vi "Simulador RLC - Versão Final - Renan_Nunes-Cardoso_Martins.vi"() -> ()   [LabVIEW 2020]
uses:
  <vilib>/Utility/file.llb/Read Delimited Spreadsheet (DBL).vi
  <vilib>/measure/NI_MABase.lvlib
panel:
  in  "?":bool
  out "?":bool
  in  "?":bool
  in  "?":u16(ring) items=["Onda Quadrada", "Onda Senoidal", "Inserir Onda"]
  in  "Plota Voltagem":bool
  in  "Plota Corrente":bool
  out "Este é um parâmetro \nescondido, serve para \nmostrar o Delta T do \narquivo insderido:":dbl
  in  "Arquivo texto da onda":path
  out "ONDA DE ENTRADA e \nVOLTAGEM NO CAPACITOR":dbl[][](graph)
  out "ONDA DE ENTRADA e CORRENTE":dbl[][](graph)
  in  "?":T1={"Taxa de Amostragem"=1000.0, "Número de amostras"=1000.0} {"Número de amostras" format="%#.6g"; "Taxa de Amostragem" format="%#.6g"}
  in  "C - Capacitância":dbl min=0.0
  in  "L -  Indutância":dbl min=0.0
  in  "R - Resistência":dbl min=0.0
  in  "Amplitude":dbl min=0.0
  in  "Duty Cicle":dbl min=0.0
  in  "Frequência":dbl min=0.0
  # "SIMULADOR RLC"
  # "LIGA/DESLIGA"
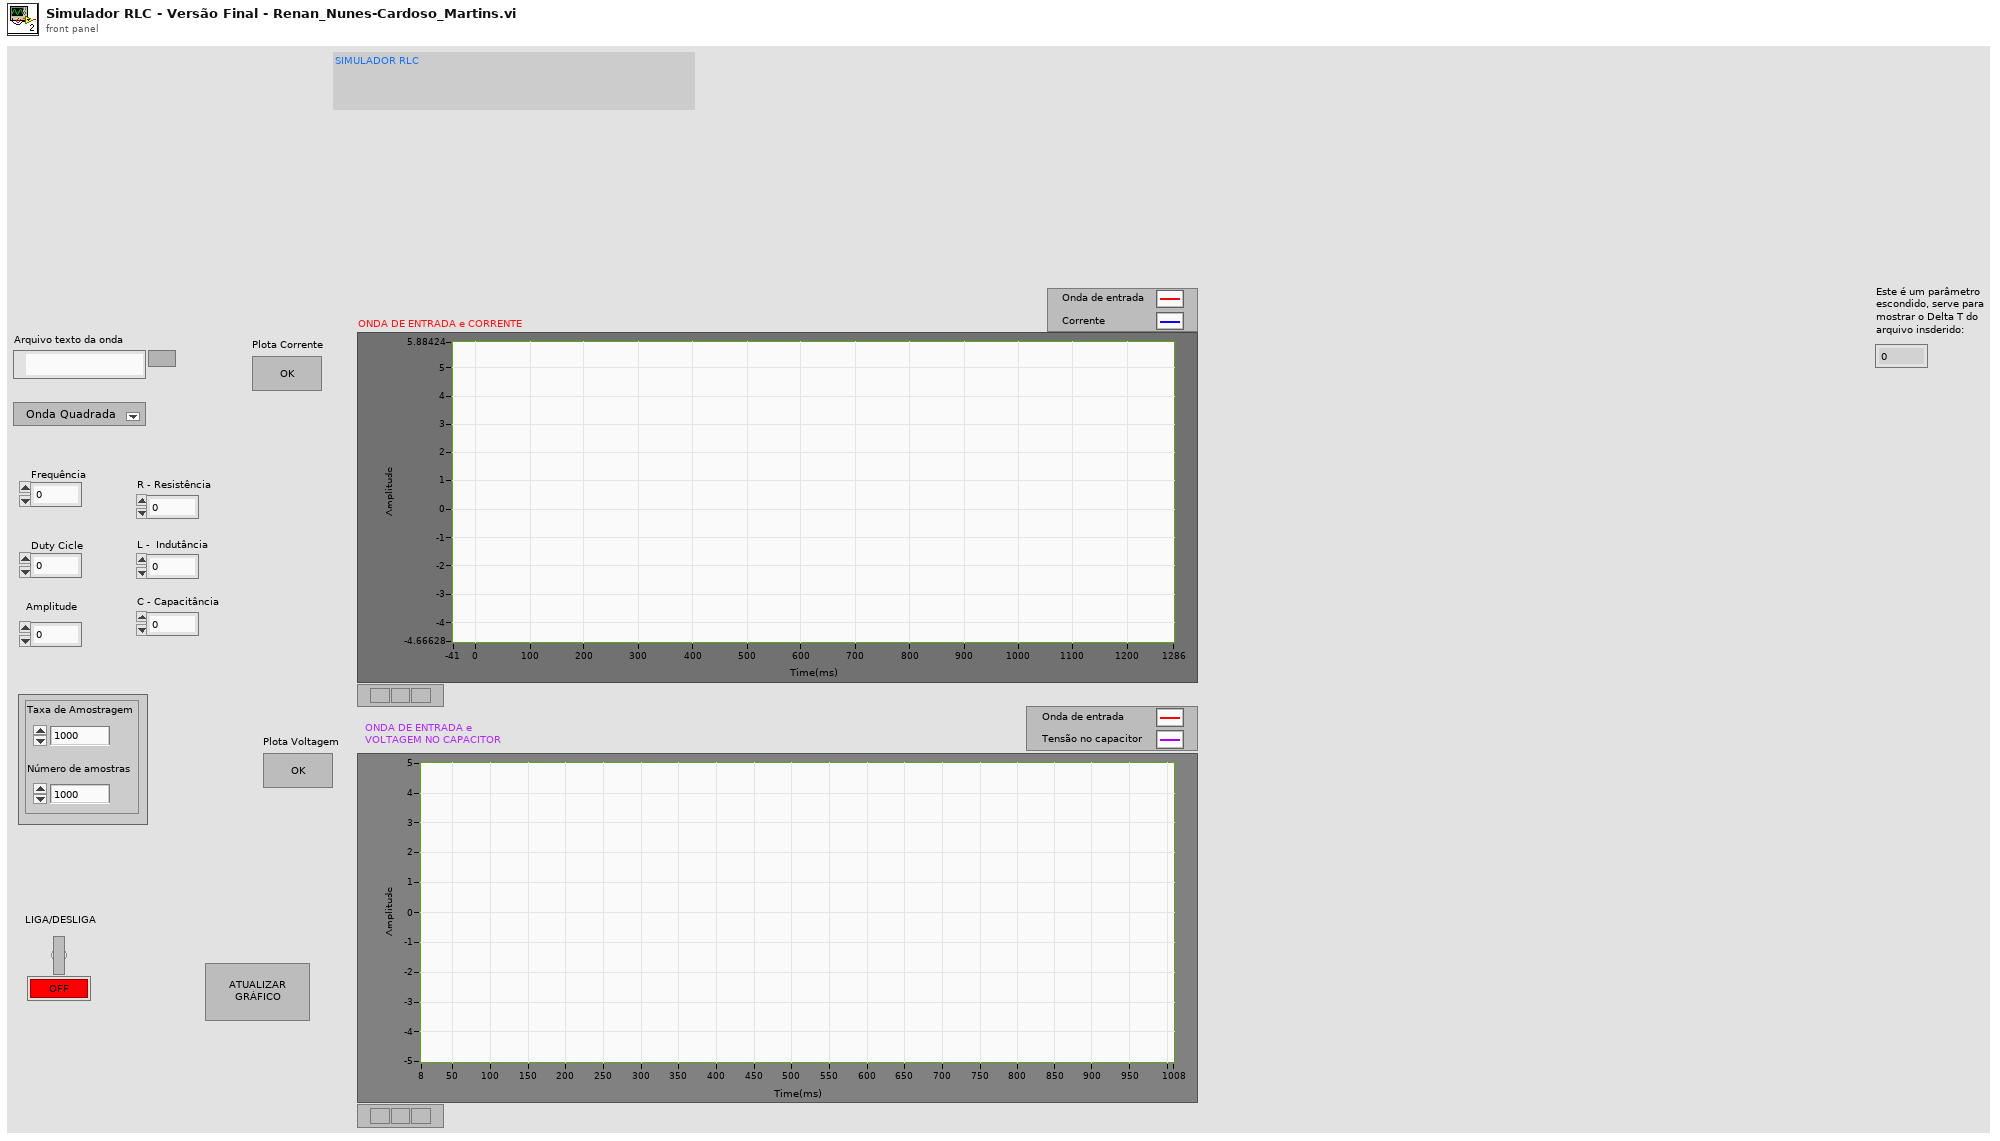
[diagram p1: front panel]
types:
  T1 = cluster{"Taxa de Amostragem":dbl, "Número de amostras":dbl}
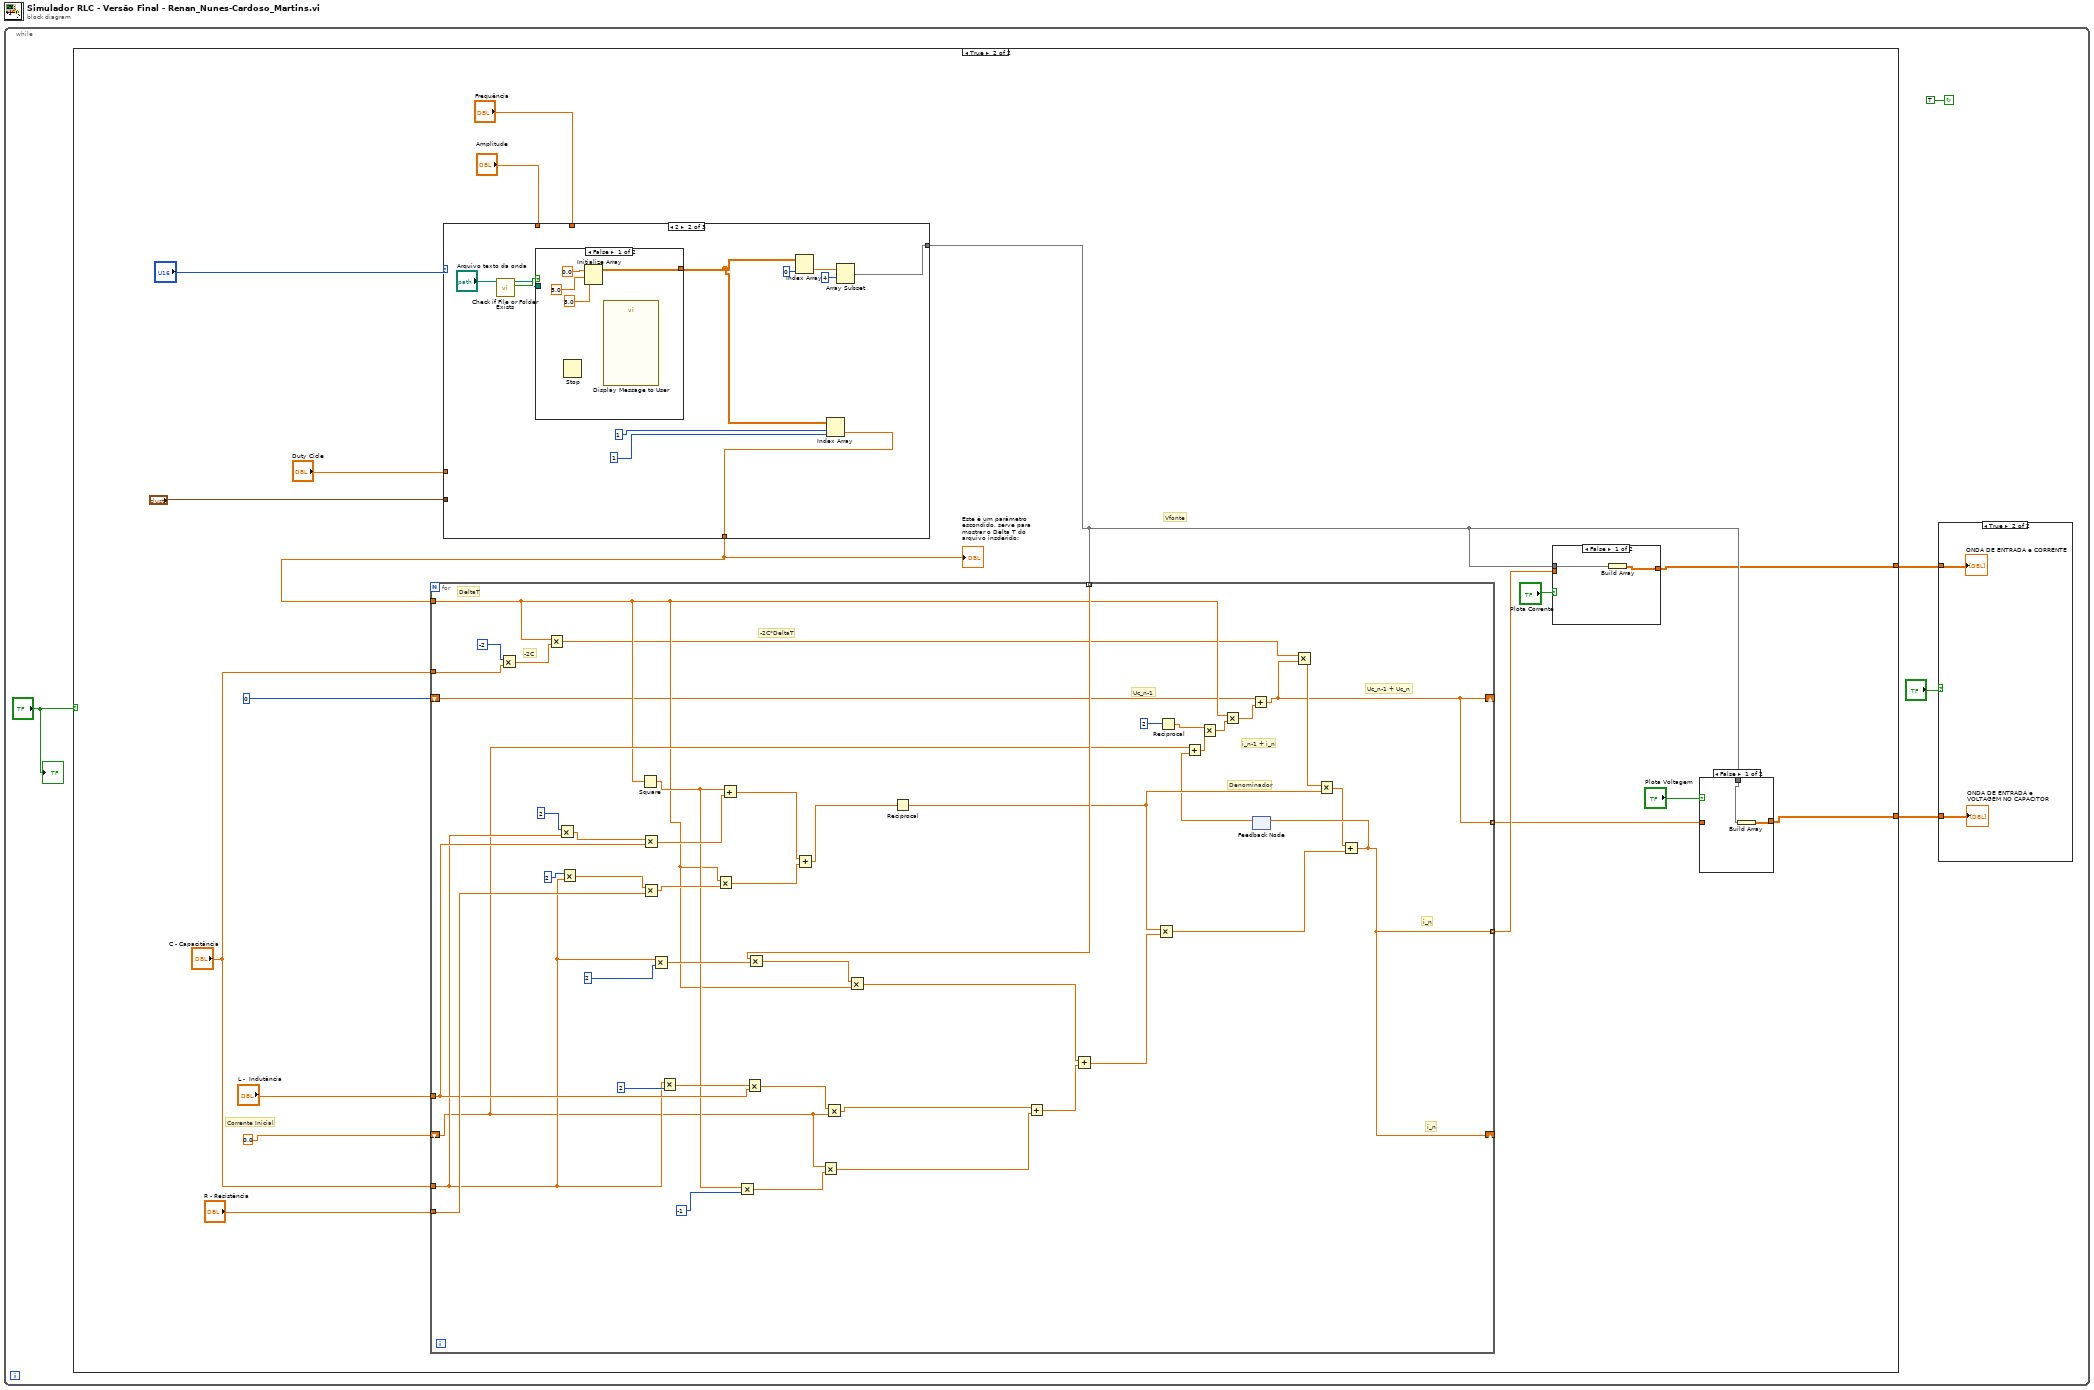
[diagram p0: block diagram]
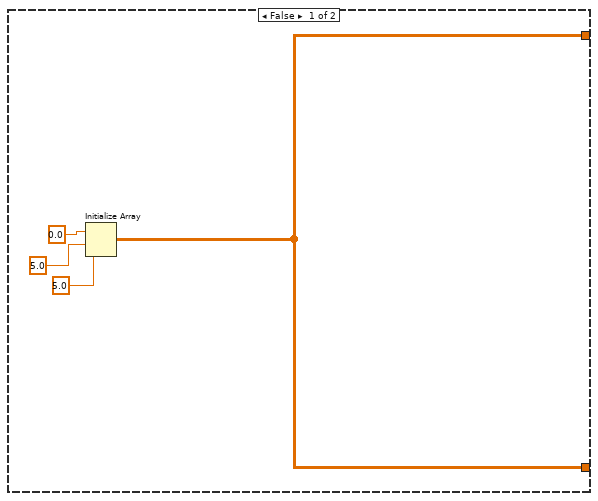
[diagram p3: hidden frame]
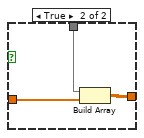
[diagram p4: hidden frame]
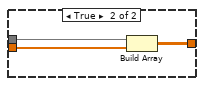
[diagram p5: hidden frame]
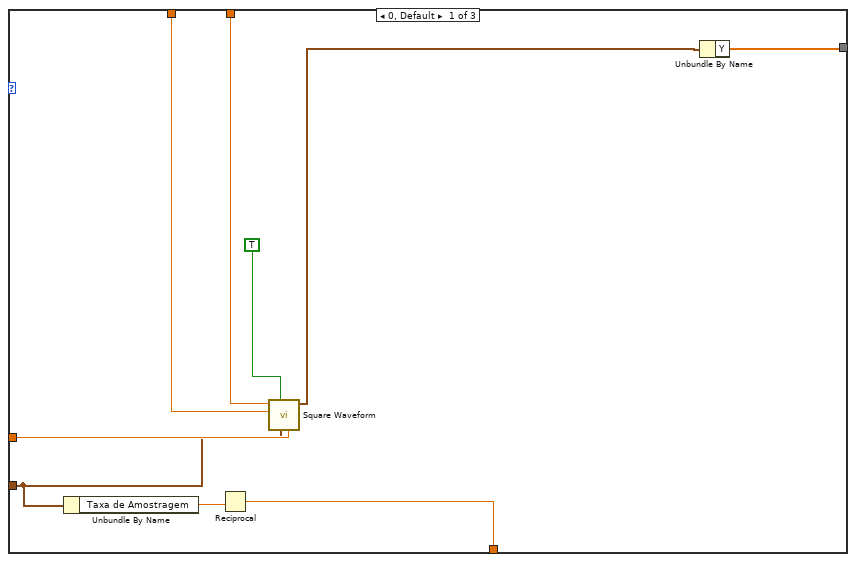
[diagram p6: hidden frame]
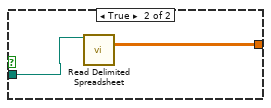
[diagram p7: hidden frame]
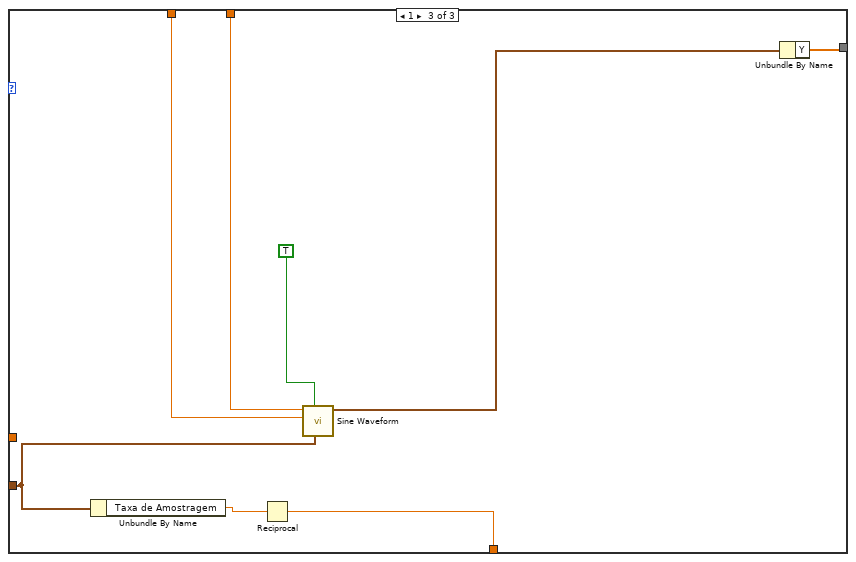
[diagram p8: hidden frame]
diagram:
  n1 = while {
    stop <- TRUE continue-if-true
    n2 = case shown="True" "?" {
      tunnel: [w8 w13] -> w3
      tunnel: [w8 w12] -> w2
      frame False {
        n3 = Initialize Array(0.0 ("element"), 5.0 ("element"), 5.0 ("element")) -> (w8:dbl[][])
      }
      frame True {
        # "Vfonte"
        # "Corrente Inicial"
        n4 = case shown="2" "?" {
          tunnel: "Amplitude" -> [w94 _ w118]
          tunnel: "Frequência" -> [w93 _ w119]
          tunnel: "Duty Cicle" -> [w92 _ _]
          tunnel: [w89 w102 w115] -> w19
          tunnel: "?" -> [w87 _ w114]
          tunnel: [w86 w98 w112] -> w17
          frame 0, Default {
            n5 = Unbundle By Name(w87) -> ("Taxa de Amostragem"=w88:dbl)
            n6 = Reciprocal(x=w88) -> (1/x=w86:dbl)
            n7 = call <vilib>:"Square Waveform.vi"("duty cycle (%)"=w92, "sampling info"=w87, "reset signal"=TRUE, "amplitude"=w94, "frequency"=w93) -> ("signal out"=w90:waveform(dbl))  [unwired: 5 in, 1 out]
            n8 = Unbundle By Name(w90) -> ("Y"=w89:dbl[])
          }
          frame 2 {
            n9 = call <vilib>:"Check if File or Folder Exists.vi"("path"="Arquivo texto da onda") -> ("file or folder exists?"=w96:bool, "dup path"=w95:path)  [unwired: 8 in, 1 out]
            n10 = case shown="False" w96 {
              tunnel: [w109 w111] -> w100
              tunnel: w95 -> [_ w110]
              frame False {
                n11 = Stop() -> ()  [unwired: 1 in]
                n12 = Initialize Array(0.0 ("element"), 5.0 ("element"), 5.0 ("element")) -> (w109:dbl[][])
                n13 = call "Display Message to User"() -> ()  [unwired: 10 in, 2 out]
              }
              frame True {
                n14 = call-poly <vilib>:"Read Delimited Spreadsheet.vi"("file path (dialog if empty)"=w110) -> ("all rows"=w111:dbl[][])  [unwired: 9 in, 5 out]
              }
            }
            n15 = Index Array(array=w100, index (col)=0 ("disabled index (col)")) -> (element=w103:dbl[])  [unwired: 1 in]
            n16 = Index Array(array=w100, index (row)=1 ("disabled index (col)"), index (col)=1 ("disabled index (col)")) -> (element=w98:dbl)
            n17 = Array Subset(array=w103, index=4) -> (w102:dbl[])  [unwired: 1 in]
          }
          frame 1 {
            n18 = Unbundle By Name(w114) -> ("Taxa de Amostragem"=w113:dbl)
            n19 = Reciprocal(x=w113) -> (1/x=w112:dbl)
            n20 = call <vilib>:"Sine Waveform.vi"("sampling info"=w114, "reset signal"=TRUE, "amplitude"=w118, "frequency"=w119) -> ("signal out"=w116:waveform(dbl))  [unwired: 6 in, 1 out]
            n21 = Unbundle By Name(w116) -> ("Y"=w115:dbl[])
          }
        }
        "Este é um parâmetro \nescondido, serve para \nmostrar o Delta T do \narquivo insderido:" <- w17
        n22 = for {
          tunnel: w19 -> [w76] mode=indexing
          tunnel: w17 -> [w50]
          tunnel: [w42] -> w21 mode=indexing
          shift-right: [w42] -> _
          shift-left: 0.0 -> [w55]
          tunnel: "R - Resistência" -> [w63]
          tunnel: "L -  Indutância" -> [w62]
          tunnel: "C - Capacitância" -> [w61]
          tunnel: "C - Capacitância" -> [w58]
          shift-right: [w40] -> _
          shift-left: 0 -> [w48]
          tunnel: [w40] -> w20 mode=indexing
          # "Uc_n-1"
          # "-2C*DeltaT"
          # "-2C"
          # "Denominador"
          # "DeltaT"
          # "i_n"
          # "i_n"
          # "Uc_n-1 + Uc_n"
          # "i_n-1 + i_n"
          n23 = Multiply(x=-2, y=w58) -> (x*y=w56:dbl)
          n24 = Multiply(x=w50, y=w56) -> (x*y=w47:dbl)
          n25 = Multiply(x=2, y=w61) -> (x*y=w84:dbl)
          n26 = Multiply(x=2, y=w61) -> (x*y=w81:dbl)
          n27 = Square(x=w50) -> (x^2=w59:dbl)
          n28 = Multiply(x=w84, y=w62) -> (x*y=w83:dbl)
          n29 = Multiply(x=w81, y=w63) -> (x*y=w80:dbl)
          n30 = Multiply(x=w61, y=2) -> (x*y=w75:dbl)
          n31 = Multiply(x=w61, y=2) -> (x*y=w72:dbl)
          n32 = Multiply(x=w50, y=w80) -> (x*y=w78:dbl)
          n33 = Add(x=w59, y=w83) -> (x+y=w79:dbl)
          n34 = Multiply(x=w59, y=-1) -> (x*y=w67:dbl)
          n35 = Multiply(x=w72, y=w62) -> (x*y=w66:dbl)
          n36 = Multiply(x=w76, y=w75) -> (x*y=w74:dbl)
          n37 = Add(x=w79, y=w78) -> (x+y=w69:dbl)
          n38 = Multiply(x=w55, y=w67) -> (x*y=w64:dbl)
          n39 = Multiply(x=w66, y=w55) -> (x*y=w65:dbl)
          n40 = Multiply(x=w74, y=w50) -> (x*y=w71:dbl)
          n41 = Reciprocal(x=w69) -> (1/x=w46:dbl)
          n42 = Add(x=w65, y=w64) -> (x+y=w70:dbl)
          n43 = Add(x=w71, y=w70) -> (x+y=w68:dbl)
          n44 = Multiply(x=w46, y=w68) -> (x*y=w44:dbl)
          n45 = Reciprocal(x=2) -> (1/x=w53:dbl)
          n46 = feedback #1() -> (w43:dbl)  [unwired: 1 in]
          n47 = Add(x=w55, y=w43) -> (x+y=w52:dbl)
          n48 = Multiply(x=w53, y=w52) -> (x*y=w51:dbl)
          n49 = Multiply(x=w50, y=w51) -> (x*y=w49:dbl)
          n50 = Add(x=w48, y=w49) -> (x+y=w40:dbl)
          n51 = Multiply(x=w47, y=w40) -> (x*y=w45:dbl)
          n52 = Multiply(x=w45, y=w46) -> (x*y=w41:dbl)
          n53 = Add(x=w41, y=w44) -> (x+y=w42:dbl)
          n54 = feedback-in #1(w42) -> ()
        }
        n55 = case shown="False" "Plota Corrente" {
          tunnel: [w35 w39] -> w12
          tunnel: w21 -> [_ w38]
          tunnel: w19 -> [w36 w37]
          frame False {
            n56 = Build Array(w36) -> (w35:dbl[][])
          }
          frame True {
            n57 = Build Array(w37, w38) -> (w39:dbl[][])
          }
        }
        n58 = case shown="False" "Plota Voltagem" {
          tunnel: [w30 w34] -> w13
          tunnel: w20 -> [_ w33]
          tunnel: w19 -> [w31 w32]
          frame False {
            n59 = Build Array(w31) -> (w30:dbl[][])
          }
          frame True {
            n60 = Build Array(w32, w33) -> (w34:dbl[][])
          }
        }
      }
    }
    n61 = case shown="True" "?" {
      tunnel: w3 -> [_ w7]
      tunnel: w2 -> [_ w6]
      frame False {
      }
      frame True {
        "ONDA DE ENTRADA e \nVOLTAGEM NO CAPACITOR" <- w7
        "ONDA DE ENTRADA e CORRENTE" <- w6
      }
    }
    "?" <- "?"
  }
